vi "RT SimpleControl.vi"(9 "HSSRPM":sgl) -> (4 "Gen Torque Demand (N m)":sgl, 5 "ColPitchDemand (Deg)":sgl)   [LabVIEW 2012]
panel:
  # "This is a minimal controller implementation provided for demonstration purposes\nPaul Fleming (1/10/13)"
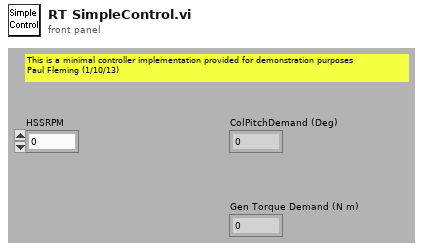
[diagram p1: front panel]
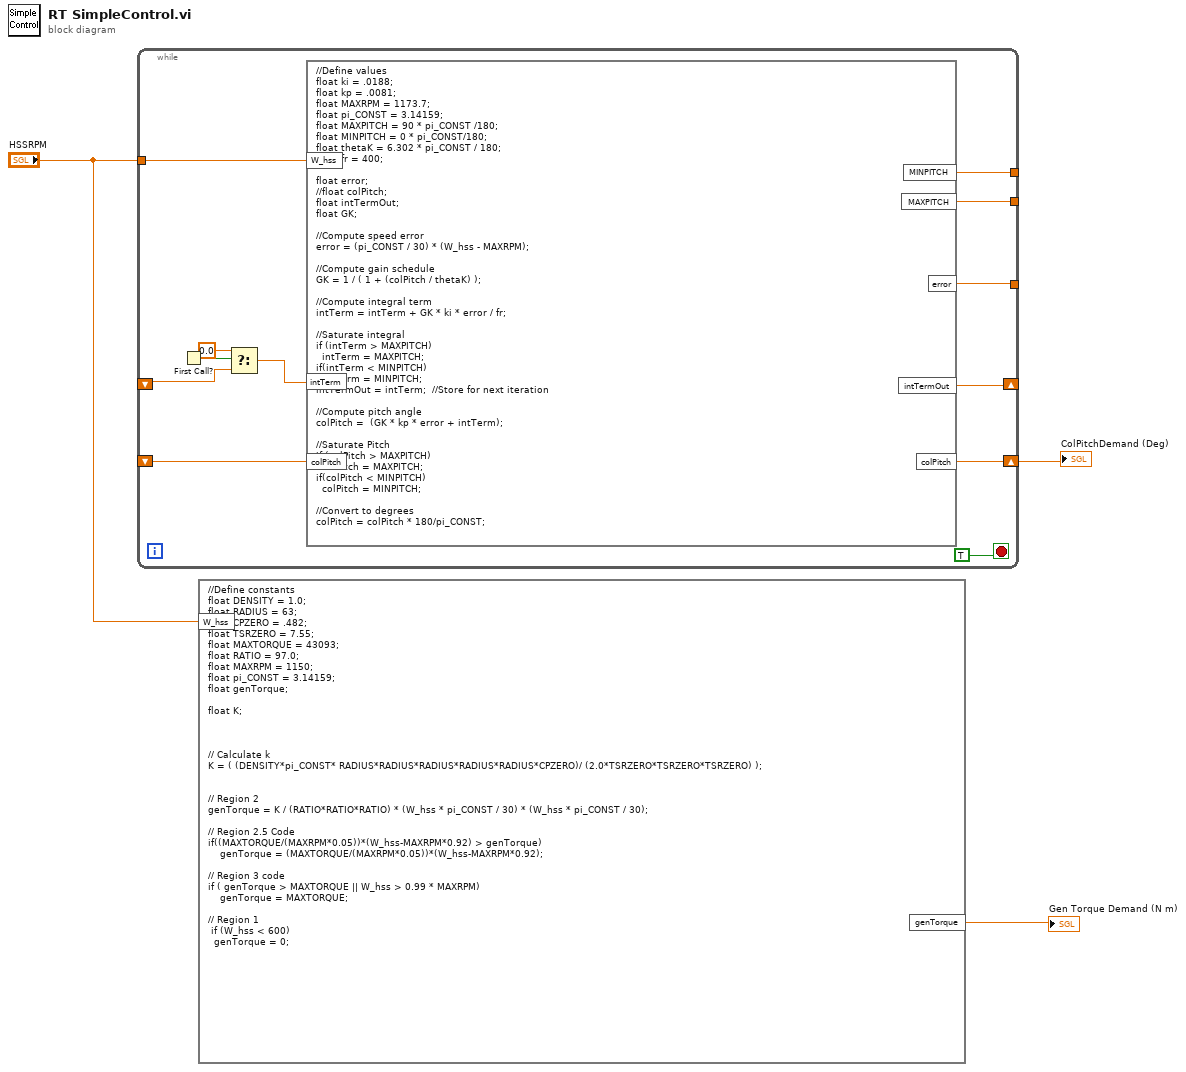
[diagram p0: block diagram]
diagram:
  n1 = while {
    tunnel: "HSSRPM" -> [w14]
    shift-right: [w12] -> _
    shift-left: _ -> [w6]
    tunnel: [w11] -> _
    tunnel: [w10] -> _
    tunnel: [w9] -> _
    shift-right: [w15] -> w2
    shift-left: _ -> [w8]
    stop <- TRUE stop-if-true
    n2 = First Call?() -> (First Call?: T/F=w7:bool)
    n3 = Select(t=0.0, s=w7, f=w6) -> (s? t:f=w4:dbl)
    n4 = formula code="//Define values\nfloat ki = .0188;\nfloat kp = .0081;\nfloat MAXRPM = 1173.7; \nfloat pi_CONST = 3.14159;\nfloat MAXPITCH = 90 * pi_CONST /180;\nfloat MINPITCH = 0 * pi_CONST/180;\nfloat thetaK = 6.302 * pi_CONST / 180;\nfloat fr = 400;\n\nfloat error;\n//float colPitch;\nfloat intTermOut;\nfloat GK;\n\n//Compute speed error\nerror = (pi_CONST / 30) * (W_hss - MAXRPM);\n\n//Compute gain schedule\nGK = 1 / ( 1 + (colPitch / thetaK) );\n\n//Compute integral term\nintTerm = intTerm + GK * ki * error / fr;\n\n//Saturate integral\nif (intTerm > MAXPITCH)\n  intTerm = MAXPITCH;\nif(intTerm < MINPITCH)\n  intTerm = MINPITCH;\nintTermOut = intTerm;  //Store for next iteration\n\n//Compute pitch angle\ncolPitch =  (GK * kp * error + intTerm);\n\n//Saturate Pitch\nif (colPitch > MAXPITCH)\n  colPitch = MAXPITCH;\nif(colPitch < MINPITCH)\n  colPitch = MINPITCH;\n\n//Convert to degrees\ncolPitch = colPitch * 180/pi_CONST;"("W_hss"=w14, "intTerm"=w4, "colPitch"=w8) -> ("colPitch"=w15:dbl, "intTermOut"=w12:dbl, "error"=w11:dbl, "MINPITCH"=w10:dbl, "MAXPITCH"=w9:dbl)
  }
  "ColPitchDemand (Deg)" <- w2
  n5 = formula code="//Define constants\nfloat DENSITY = 1.0; \nfloat RADIUS = 63;\nfloat CPZERO = .482;\nfloat TSRZERO = 7.55; \nfloat MAXTORQUE = 43093;\nfloat RATIO = 97.0;\nfloat MAXRPM = 1150; \nfloat pi_CONST = 3.14159;\nfloat genTorque;\n\nfloat K; \n\n\n\n// Calculate k\nK = ( (DENSITY*pi_CONST* RADIUS*RADIUS*RADIUS*RADIUS*RADIUS*CPZERO)/ (2.0*TSRZERO*TSRZERO*TSRZERO) );\n\n\n// Region 2\ngenTorque = K / (RATIO*RATIO*RATIO) * (W_hss * pi_CONST / 30) * (W_hss * pi_CONST / 30);\n\n// Region 2.5 Code\nif((MAXTORQUE/(MAXRPM*0.05))*(W_hss-MAXRPM*0.92) > genTorque)\n    genTorque = (MAXTORQUE/(MAXRPM*0.05))*(W_hss-MAXRPM*0.92);\n\n// Region 3 code\nif ( genTorque > MAXTORQUE || W_hss > 0.99 * MAXRPM)\n    genTorque = MAXTORQUE;\n\n// Region 1\n if (W_hss < 600)\n  genTorque = 0;"("W_hss"="HSSRPM") -> ("genTorque"=→"Gen Torque Demand (N m)":dbl)
